vi "Beam.vi"(8 "shiftY":dbl, 9 "shiftX":dbl) -> (0 "Rate":dbl=12800.0, 2 "Scanners trajectories":dbl[][](graph), 3 "XY Graph":cluster{"sine wave":dbl[], "sine wave":dbl[]}(graph)={"sine wave"=[0.0, 0.0012266918581854505, 0.0024504285082390153, 0.003668261861384044, 0.0048772580504032065, 0.006074504497581597, 0.007257116931361559, 0.0084222463348055, 0.009567085809127244, 0.010688877335757052, 0.01178491842064994, 0.012852568604830542, 0.013889255825490054, 0.014892482612310833, 0.015859832104091136, 0.01678897387117546, 0.017677669529663688, 0.01852377813387398, 0.019325261334068422, 0.020080188287016125, 0.02078674030756363, 0.021443215250006805, 0.022048031608708874, 0.022599732328086087, 0.023096988312782167, 0.023538601629575523, 0.023923508393305218, 0.024250781329863604, 0.02451963201008076, 0.02472941274911953, 0.02487961816680492, 0.024969886405129316, 0.024999999999999998, 0.024969886405129316, 0.02487961816680492, 0.02472941274911953, 0.02451963201008076, 0.024250781329863604, 0.023923508393305218, 0.023538601629575523, 0.023096988312782164, 0.022599732328086087, 0.02204803160870887, 0.021443215250006805, 0.020786740307563625, 0.020080188287016125, 0.01932526133406842, 0.01852377813387398, 0.017677669529663684, 0.01678897387117546, 0.015859832104091136, 0.014892482612310833, 0.013889255825490054, 0.012852568604830542, 0.01178491842064994, 0.01068887733575705, 0.009567085809127244, 0.008422246334805499, 0.007257116931361559, 0.0060745044975815945, 0.0048772580504032065, 0.0036682618613840404, 0.002450428508239015, 0.0012266918581854466, 0.0, -0.0012266918581854548, -0.002450428508239015, -0.0036682618613840486, -0.0048772580504032065, -0.006074504497581602, -0.007257116931361558, -0.008422246334805508, -0.009567085809127244, -0.010688877335757059, -0.01178491842064994, -0.01285256860483055, -0.013889255825490054, -0.014892482612310841, -0.015859832104091136, -0.016788973871175467, -0.017677669529663684, -0.018523778133873986, -0.01932526133406842, -0.020080188287016132, -0.020786740307563625, -0.021443215250006812, -0.02204803160870887, -0.022599732328086094, -0.023096988312782164, -0.02353860162957553, -0.023923508393305218, -0.02425078132986361, -0.02451963201008076, -0.024729412749119536, -0.02487961816680492, -0.024969886405129323, -0.024999999999999998, -0.024969886405129323, -0.02487961816680492, -0.024729412749119536, -0.02451963201008076, -0.02425078132986361, -0.023923508393305218, -0.02353860162957553, -0.023096988312782164, -0.022599732328086094, -0.02204803160870887, -0.021443215250006812, -0.020786740307563625, -0.020080188287016132, -0.01932526133406842, -0.018523778133873986, -0.017677669529663684, -0.016788973871175467, -0.015859832104091136, -0.01489248261231084, -0.013889255825490054, -0.012852568604830547, -0.01178491842064994, -0.010688877335757054, -0.009567085809127244, -0.0084222463348055, -0.007257116931361559, -0.0060745044975815945, -0.0048772580504032065, -0.003668261861384039, -0.002450428508239015, -0.0012266918581854435], "sine wave"=[0.025, 0.024969886405129312, 0.024879618166804923, 0.024729412749119526, 0.024519632010080762, 0.0242507813298636, 0.02392350839330522, 0.02353860162957552, 0.023096988312782167, 0.022599732328086083, 0.022048031608708874, 0.0214432152500068, 0.02078674030756363, 0.02008018828701612, 0.019325261334068422, 0.018523778133873976, 0.017677669529663688, 0.016788973871175457, 0.015859832104091136, 0.01489248261231083, 0.013889255825490054, 0.012852568604830542, 0.01178491842064994, 0.01068887733575705, 0.009567085809127244, 0.008422246334805499, 0.007257116931361558, 0.006074504497581595, 0.004877258050403205, 0.003668261861384042, 0.0024504285082390127, 0.0012266918581854487, -3.0357660829594124e-18, -0.0012266918581854518, -0.0024504285082390187, -0.003668261861384045, -0.004877258050403211, -0.006074504497581599, -0.0072571169313615635, -0.008422246334805502, -0.009567085809127249, -0.010688877335757054, -0.011784918420649947, -0.012852568604830543, -0.013889255825490061, -0.014892482612310833, -0.015859832104091143, -0.016788973871175457, -0.017677669529663695, -0.018523778133873972, -0.01932526133406843, -0.020080188287016118, -0.020786740307563636, -0.021443215250006798, -0.02204803160870888, -0.02259973232808608, -0.023096988312782174, -0.023538601629575516, -0.023923508393305225, -0.024250781329863597, -0.024519632010080766, -0.024729412749119523, -0.024879618166804927, -0.02496988640512931, -0.025, -0.02496988640512931, -0.024879618166804923, -0.024729412749119523, -0.024519632010080762, -0.024250781329863597, -0.02392350839330522, -0.023538601629575516, -0.023096988312782167, -0.02259973232808608, -0.022048031608708874, -0.021443215250006798, -0.02078674030756363, -0.020080188287016118, -0.019325261334068422, -0.018523778133873972, -0.017677669529663684, -0.016788973871175457, -0.015859832104091132, -0.01489248261231083, -0.01388925582549005, -0.012852568604830542, -0.011784918420649933, -0.010688877335757052, -0.009567085809127235, -0.0084222463348055, -0.00725711693136155, -0.006074504497581597, -0.004877258050403196, -0.003668261861384044, -0.0024504285082390044, -0.0012266918581854505, 1.0842021724855044e-17, 0.00122669185818545, 0.002450428508239026, 0.0036682618613840434, 0.004877258050403218, 0.006074504497581597, 0.00725711693136157, 0.0084222463348055, 0.009567085809127256, 0.010688877335757052, 0.011784918420649953, 0.012852568604830542, 0.013889255825490067, 0.01489248261231083, 0.01585983210409115, 0.016788973871175457, 0.017677669529663702, 0.018523778133873972, 0.019325261334068436, 0.020080188287016118, 0.020786740307563643, 0.021443215250006798, 0.022048031608708888, 0.02259973232808608, 0.02309698831278218, 0.023538601629575516, 0.02392350839330523, 0.024250781329863597, 0.02451963201008077, 0.024729412749119523, 0.02487961816680493, 0.02496988640512931]})   [LabVIEW 2021]
uses:
  <vilib>/Analysis/NI_AALBase.lvlib
panel:
  out "Cycle duration":i32=128
  in  "Number of cycles":i32=20
  # "Przy 12800 S/s i 128 sampli na bodziec, czas trwania 1 cyklu 10 ms"
  # "przerwa ustawiona na 600 ms"
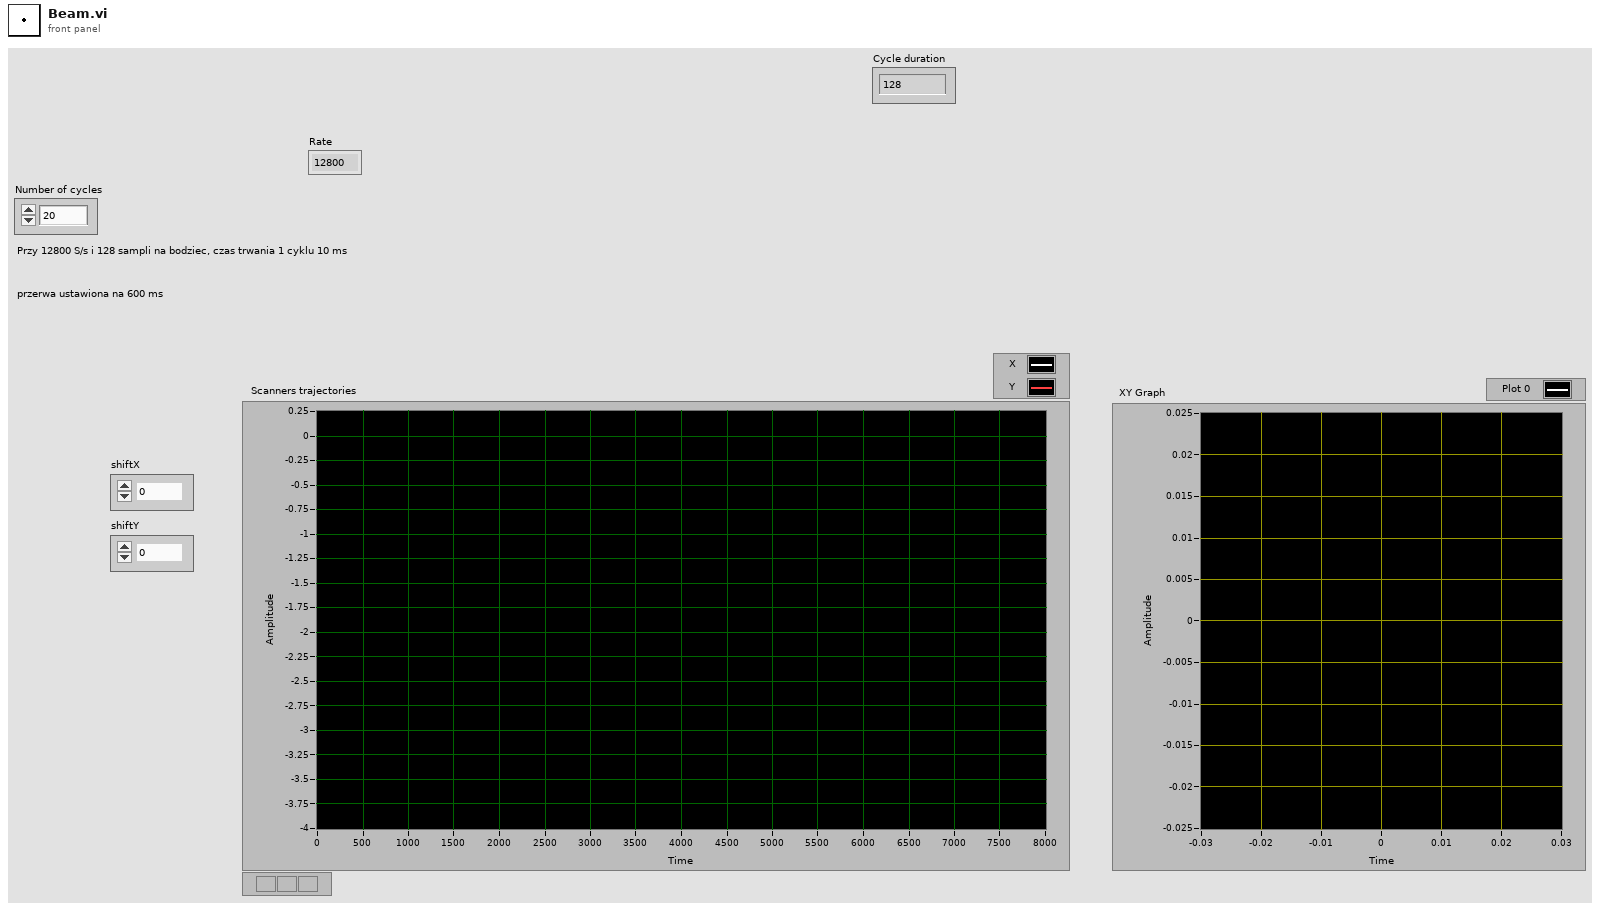
[diagram p1: front panel]
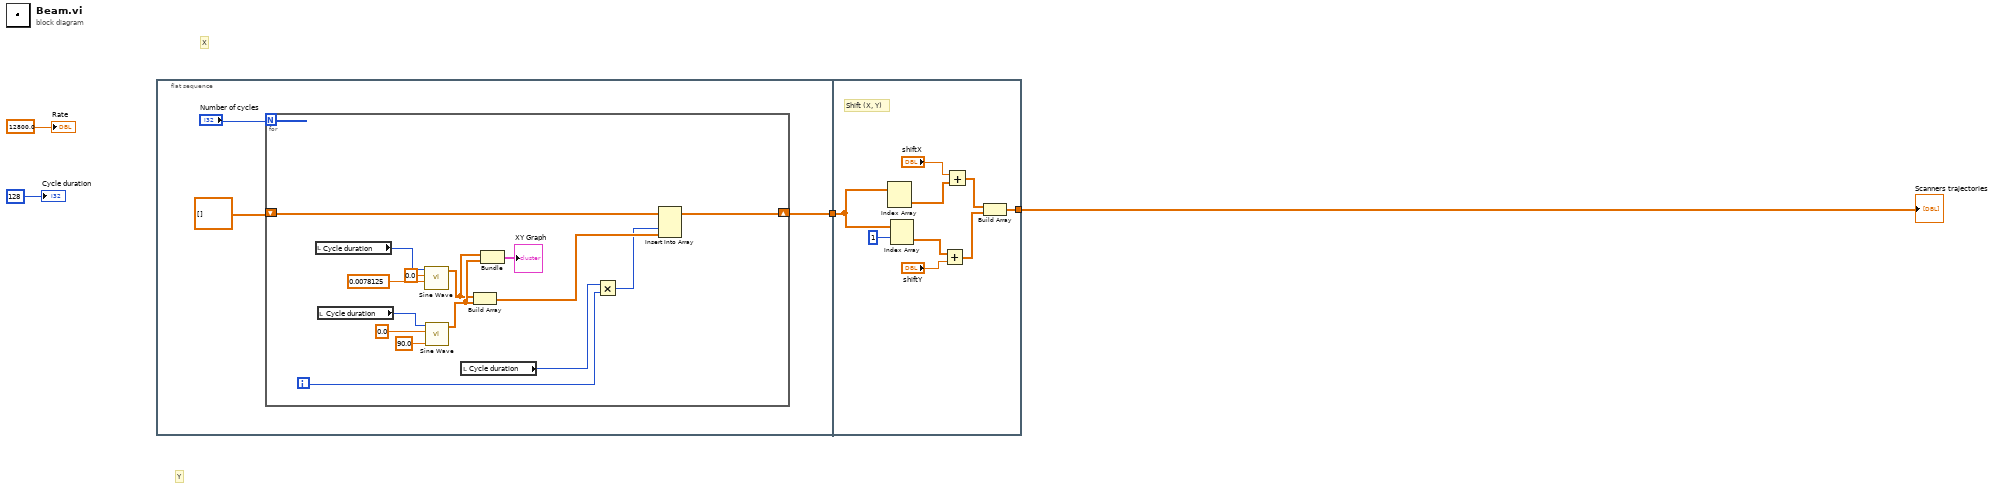
[diagram p0: block diagram]
diagram:
  # "Y"
  # "X"
  n1 = flat-sequence {
    tunnel: [w5] -> w1
    tunnel: [w31] -> w4
    tunnel: w1 -> [w23]
    frame #0 {
      n2 = for {
        N: "Number of cycles" -> [_]
        shift-right: [w18] -> w5
        shift-left: dbl[][] [] -> [w20]
        i -> [w16]
        n3 = local read "Cycle duration"() -> (w15:i32)
        n4 = local read "Cycle duration"() -> (w14:i32)
        n5 = call <vilib>:"Sine Wave.vi"("samples"=w15, "amplitude"=0.0, "frequency"=0.0078125) -> ("sine wave"=w11:dbl[])  [unwired: 2 in, 2 out]
        n6 = call <vilib>:"Sine Wave.vi"("samples"=w14, "amplitude"=0.0, "phase in"=90.0) -> ("sine wave"=w12:dbl[])  [unwired: 2 in, 2 out]
        n7 = local read "Cycle duration"() -> (w13:i32)
        n8 = Build Array(w11, w12) -> (w19:dbl[][])
        n9 = Bundle("sine wave"=w11, "sine wave"=w12) -> (→"XY Graph":cluster{"sine wave":dbl[], "sine wave":dbl[]})  [unwired: 1 in]
        n10 = Multiply(x=w13, y=w16) -> (x*y=w17:i32)
        n11 = Insert Into Array(array=w20, index (col)=w17, new element=w19) -> (w18:dbl[][])  [unwired: 1 in]
      }
    }
    frame #1 {
      # "Shift (X, Y)"
      n12 = Index Array(array=w23) -> (element=w29:dbl[])  [unwired: 2 in]
      n13 = Index Array(array=w23, index (row)=1) -> (element=w28:dbl[])  [unwired: 1 in]
      n14 = Add(x=w28, y="shiftY") -> (x+y=w25:dbl[])
      n15 = Add(x="shiftX", y=w29) -> (x+y=w26:dbl[])
      n16 = Build Array(w26, w25) -> (w31:dbl[][])
    }
  }
  "Scanners trajectories" <- w4
  "Rate" <- 12800.0 ("Rate")
  "Cycle duration" <- 128
